vi "Write PressureTransducerCompensator.vi"(10 "PressureTransducerCompensator.lvclass":refnum<class "PressureTransducerCompensator.lvclass">, 11 "DualActingPneumaticCylinder in":refnum<class "DualActingPneumaticCylinder.lvclass">) -> (3 "DualActingPneumaticCylinder out":refnum<class "DualActingPneumaticCylinder.lvclass">)   [LabVIEW 2013, in "DualActingPneumaticCylinder.lvclass"]
uses:
  DualActingPneumaticCylinder.lvclass
  PressureTransducerCompensator/PressureTransducerCompensator.lvclass
  DualActingPneumaticCylinder.lvclass/DualActingPneumaticCylinder.ctl
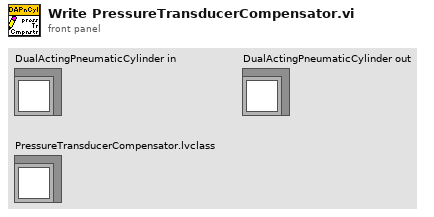
[diagram p1: front panel]
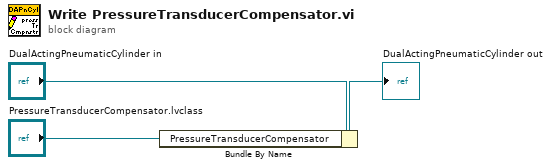
[diagram p0: block diagram]
diagram:
  n1 = Bundle By Name(cluster="DualActingPneumaticCylinder in", "PressureTransducerCompensator"="PressureTransducerCompensator.lvclass") -> (→"DualActingPneumaticCylinder out":refnum<class "DualActingPneumaticCylinder.lvclass">)
